vi "GetModuleName.vi"(4 "error in (no error)":errorcluster, 6 "hModule (0)":i32, 7 "hProcess (0)":i32) -> (0 "error out":errorcluster, 2 "Full Module Name":string, 3 "Module Name":string)   [LabVIEW 2011]
uses:
  psapi.dll
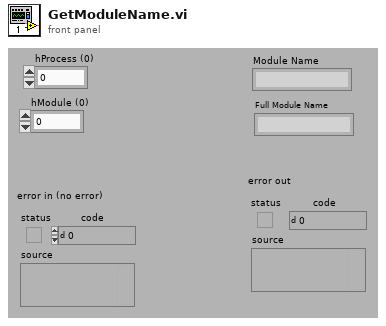
[diagram p1: front panel]
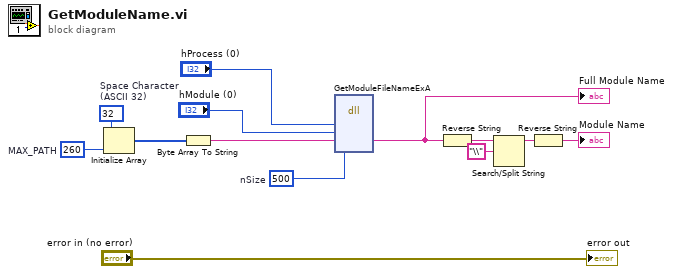
[diagram p0: block diagram]
diagram:
  w2 = 260  # MAX_PATH
  w10 = u8 32  # Space Character (ASCII 32)
  w7 = 500  # nSize
  n1 = Initialize Array(w10, w2) -> (w8:u8[])
  n2 = Byte Array To String(unsigned byte array=w8) -> (string=w9:string)
  n3 = dll-call lib="psapi.dll" fn="GetModuleFileNameExA"("hProcess"="hProcess (0)", "hModule"="hModule (0)", "ModuleName"=w9, "nSize"=w7) -> ("ModuleName"=w6:string)  [unwired: 6 in, 3 out]
  "Full Module Name" <- w6
  n4 = Reverse String(1:w6) -> (0:w11:string)
  n5 = Search/Split String(string=w11, search string/char (-)="\\") -> (substring before match=w13:string)  [unwired: 3 out]
  n6 = Reverse String(1:w13) -> (0:→"Module Name":string)
  "error out" <- "error in (no error)"
